vi "KH_DAQ_TURCK_ScaleAI.vi"(8 "Messwert Turck":i16[](array[numeric]), 10 "EIP_AI":T1 {"Offset" format="%.4f"; "Phys Max" format="%.4f"; "Phys Min" format="%.4f"}, 11 "Nr.":i32) -> (3 "Messwert skaliert":sgl[](array[numeric]))   [LabVIEW 2021]
uses:
  KH_DAQ_TypeDefs_Cluster AI.ctl
  KH_DAQ_TypeDefs_Messbereich.ctl
  KH EthernetIPConfig 17.14/KH EthernetIPConfig TypeDefs ModuleTyp.ctl
  KH_DAQ_TypeDefs_Bereich.ctl
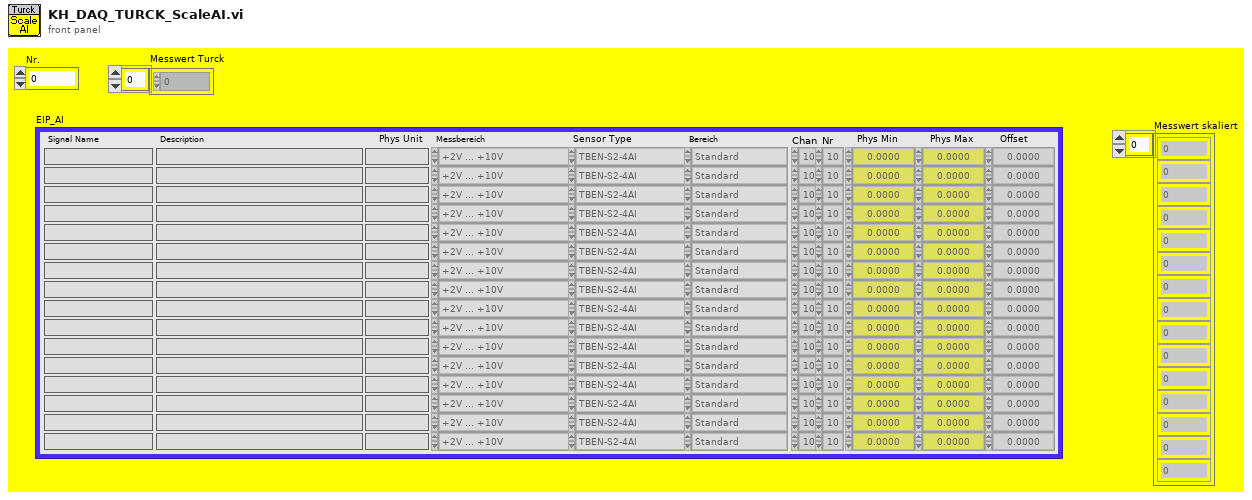
[diagram p1: front panel]
types:
  T1 = typedef "KH_DAQ_TypeDefs_Cluster AI.ctl" = cluster{"Signal Name":string[], "Description":string[], "Phys Unit":string[], "Messbereich":T2[], "Chan":u16[], "Phys Min":sgl[], "Phys Max":sgl[], "Offset":sgl[], "Nr":u16[], "SensorType 2":T3[], "Bereich":T4[]}
  T2 = typedef "KH_DAQ_TypeDefs_Messbereich.ctl" = enum16{"-10V ... +10V", "0V ... +10V", "+2V ... +10V", "0V ... +5V", "+1V ... +5V", "-1V ... +1V", "-500mV ... +500mV", "-100mV ... +100mV", "-50mV ... +50mV", "0mA ... +20mA", "+4mA ... +20mA", "-20mA ... +20mA", "0 Ohm ... 100 Ohm", "0 Ohm ... 400 Ohm", "0 Ohm ... 2000 Ohm", "0 Ohm ... 4000 Ohm", "-200°C ... 150°C PT100", "-200°C ... 150°C PT200", "-200°C ... 150°C PT500", "-200°C ... 150°C PT1000", "-60°C ... 150°C Ni100", "-60°C ... 150°C Ni1000", "-200°C ... 850°C PT100", "-200°C ... 850°C PT200", "-200°C ... 850°C PT500", "-200°C ... 850°C PT1000", "-50°C ... 250°C Ni100", "-50°C ... 250° Ni 1000"}
  T3 = typedef "KH EthernetIPConfig TypeDefs ModuleTyp.ctl" = enum16{"TBEN-S2-4AI", "TBEN-S1-8DXP", "TBEN-S2-2RFID-4DXP", "TBEN-S2-4AO", "TBEN-S2-4IOL"}
  T4 = typedef "KH_DAQ_TypeDefs_Bereich.ctl" = enum16{"Standard", "extended Range", "NE43", ""}
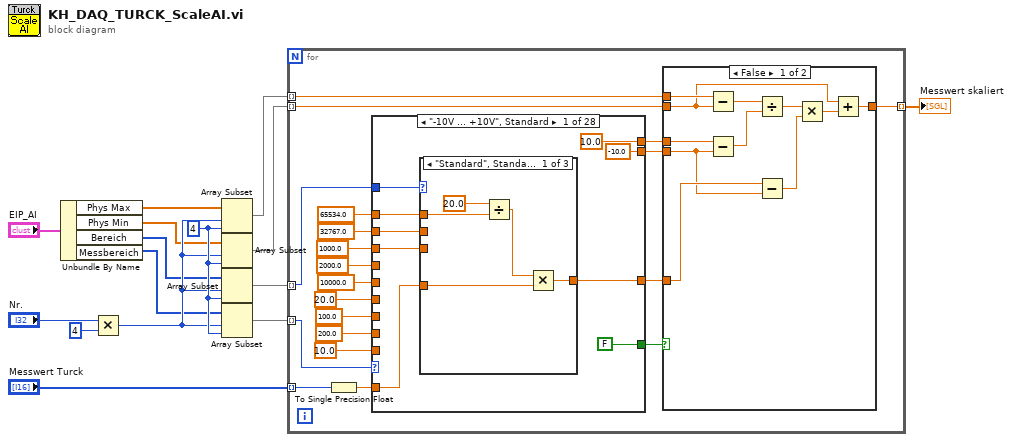
[diagram p0: block diagram]
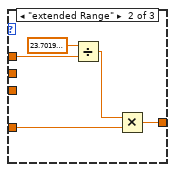
[diagram p3: hidden frame]
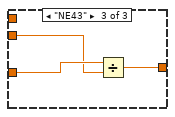
[diagram p4: hidden frame]
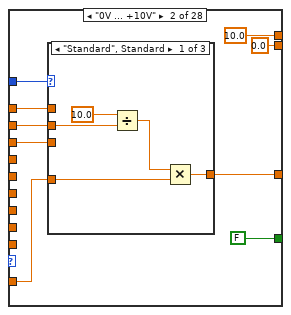
[diagram p5: hidden frame]
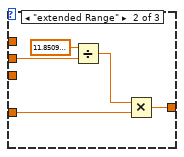
[diagram p6: hidden frame]
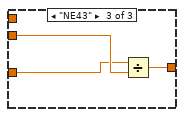
[diagram p7: hidden frame]
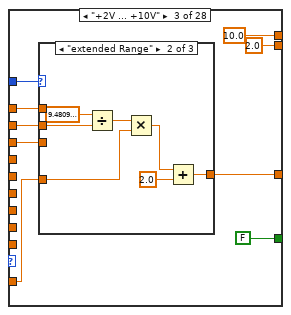
[diagram p8: hidden frame]
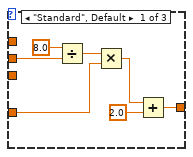
[diagram p9: hidden frame]
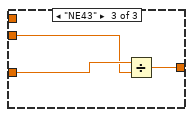
[diagram p10: hidden frame]
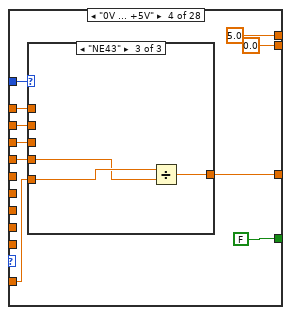
[diagram p11: hidden frame]
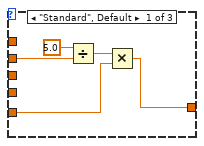
[diagram p12: hidden frame]
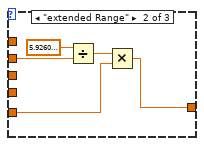
[diagram p13: hidden frame]
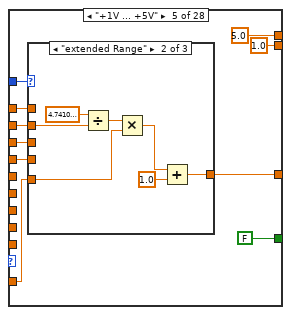
[diagram p14: hidden frame]
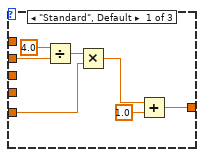
[diagram p15: hidden frame]
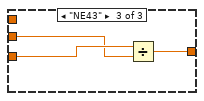
[diagram p16: hidden frame]
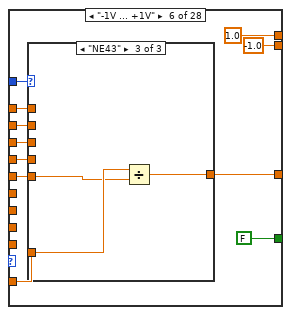
[diagram p17: hidden frame]
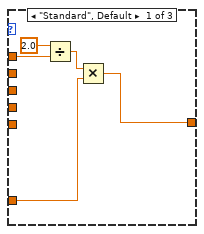
[diagram p18: hidden frame]
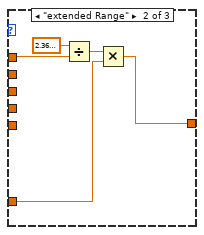
[diagram p19: hidden frame]
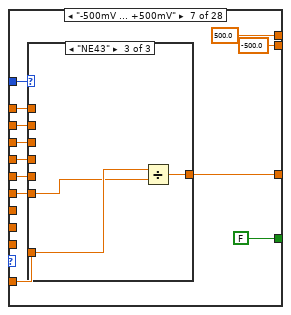
[diagram p20: hidden frame]
diagram:
  w15 = 4 ("length")
  n1 = Unbundle By Name("EIP_AI") -> ("Phys Max"=w8:sgl[], "Phys Min"=w9:sgl[], "Bereich"=w10:T4[], "Messbereich"=w11:T2[])
  n2 = Multiply(x="Nr.", y=4) -> (x*y=w14:i32)
  n3 = Array Subset(array=w8, index=w14, length=w15) -> (w7:sgl[])
  n4 = Array Subset(array=w9, index=w14, length=w15) -> (w6:sgl[])
  n5 = Array Subset(array=w10, index=w14, length=w15) -> (w5:T4[])
  n6 = Array Subset(array=w11, index=w14, length=w15) -> (w4:T2[])
  n7 = for {
    tunnel: [w22] -> w1 mode=indexing
    tunnel: w7 -> [w20] mode=indexing
    tunnel: w6 -> [w19] mode=indexing
    tunnel: w5 -> [w18] mode=indexing
    tunnel: w4 -> [w17] mode=indexing
    tunnel: "Messwert Turck" -> [w16] mode=indexing
    n8 = To Single Precision Float(number=w16) -> (single precision float=w32:sgl)
    n9 = case shown="\"-10V ... +10V\", Standard" w17 {
      tunnel: w18 -> [w56 w78 w100 w127 w150 w178 w203 w229 w256 w283 w310 w341 _ _ _ _ _ _ _ _ _ _ _ _ _ _ _ _]
      tunnel: sgl 65534.0 ("Sollwert 2") -> [w55 w77 w99 w126 w149 w177 w202 w228 w255 w282 w309 w340 _ _ _ _ _ _ _ _ _ _ _ _ _ _ _ _]
      tunnel: sgl 32767.0 ("Sollwert 2") -> [w54 w76 w98 w125 w148 w176 w201 w227 w254 w281 w308 w339 w362 w370 w378 w386 _ _ _ _ _ _ _ _ _ _ _ _]
      tunnel: sgl 1000.0 ("Sollwert 2") -> [w53 w75 w97 w124 w147 w175 w200 w226 w253 w280 w307 w338 _ _ _ _ _ _ _ _ _ _ _ _ _ _ _ _]
      tunnel: w32 -> [w52 w74 w96 w123 w146 w174 w199 w225 w252 w279 w306 w337 w361 w369 w377 w385 w390 w394 w398 w402 w406 w410 w414 w418 w422 w426 w430 w434]
      tunnel: [w51 w73 w95 w122 w145 w173 w198 w224 w251 w278 w305 w336 w360 w368 w376 w384 w389 w393 w397 w401 w405 w409 w412 w417 w421 w425 w429 w433] -> w23
      tunnel: sgl 2000.0 ("Sollwert 2") -> [_ _ _ w121 w144 w172 w197 w223 w250 w277 w304 w335 _ _ _ _ _ _ _ _ _ _ _ _ _ _ _ _]
      tunnel: sgl 10000.0 ("Sollwert 2") -> [_ _ _ _ _ w171 w196 w222 w249 w276 w303 w334 _ _ _ _ _ _ _ _ _ _ _ _ _ _ _ _]
      tunnel: sgl 20.0 ("Sollwert 2") -> [_ _ _ _ _ _ w195 w221 w248 w275 w302 w333 _ _ _ _ _ _ _ _ _ _ _ _ _ _ _ _]
      tunnel: sgl 100.0 ("Sollwert 2") -> [_ _ _ _ _ _ _ w220 w247 w274 w301 w332 _ _ _ _ w388 w392 w396 w400 w404 w408 _ _ _ _ _ _]
      tunnel: sgl 200.0 ("Sollwert 2") -> [_ _ _ _ _ _ _ _ w246 w273 w300 w331 _ _ _ _ _ _ _ _ _ _ _ _ _ _ _ _]
      tunnel: sgl 10.0 ("Sollwert 2") -> [_ _ _ _ _ _ _ _ _ _ _ _ _ _ _ _ _ _ _ _ _ _ w413 w416 w420 w424 w428 w432]
      tunnel: [sgl -10.0 ("Messwert 2") sgl 0.0 ("Messwert 2") sgl 2.0 ("Messwert 2") sgl 0.0 ("Messwert 2") sgl 1.0 ("Messwert 2") sgl -1.0 ("Messwert 2") sgl -500.0 ("Messwert 2") sgl -100.0 ("Messwert 2") sgl -50.0 ("Messwert 2") sgl 0.0 ("Messwert 2") sgl 4.0 ("Messwert 2") sgl -20.0 ("Messwert 2") sgl 0.0 ("Messwert 2") sgl 0.0 ("Messwert 2") sgl 0.0 ("Messwert 2") sgl 0.0 ("Messwert 2") _ _ _ _ _ _ _ _ _ _ _ _] -> w25
      tunnel: [sgl 10.0 ("Messwert 2") sgl 10.0 ("Messwert 2") sgl 10.0 ("Messwert 2") sgl 5.0 ("Messwert 2") sgl 5.0 ("Messwert 2") sgl 1.0 ("Messwert 2") sgl 500.0 ("Messwert 2") sgl 100.0 ("Messwert 2") sgl 50.0 ("Messwert 2") sgl 20.0 ("Messwert 2") sgl 20.0 ("Messwert 2") sgl 20.0 ("Messwert 2") sgl 100.0 ("Messwert 2") sgl 400.0 ("Messwert 2") sgl 2000.0 ("Messwert 2") sgl 4000.0 ("Messwert 2") _ _ _ _ _ _ _ _ _ _ _ _] -> w24
      tunnel: [FALSE FALSE FALSE FALSE FALSE FALSE FALSE FALSE FALSE FALSE FALSE FALSE FALSE FALSE FALSE FALSE TRUE TRUE TRUE TRUE TRUE TRUE TRUE TRUE TRUE TRUE TRUE TRUE] -> w21
      frame "-10V ... +10V", Default {
        n10 = case shown="\"Standard\", Standard" w56 {
          tunnel: w55 -> [w60 w65 _]
          tunnel: w54 -> [_ _ _]
          tunnel: w53 -> [_ _ w68]
          tunnel: w52 -> [w59 w64 w69]
          tunnel: [w57 w62 w67] -> w51
          frame "Standard", Default {
            n11 = Divide(x=sgl 20.0 ("Messwert 2"), y=w60) -> (x/y=w58:sgl)
            n12 = Multiply(x=w58, y=w59) -> (x*y=w57:sgl)
          }
          frame "extended Range" {
            n13 = Divide(x=sgl 23.702 ("Messwert 2"), y=w65) -> (x/y=w63:sgl)
            n14 = Multiply(x=w63, y=w64) -> (x*y=w62:sgl)
          }
          frame "NE43" {
            n15 = Divide(x=w69, y=w68) -> (x/y=w67:sgl)
          }
        }
      }
      frame "0V ... +10V" {
        n16 = case shown="\"Standard\", Standard" w78 {
          tunnel: w77 -> [_ _ _]
          tunnel: w76 -> [w79 w84 _]
          tunnel: w75 -> [_ _ w91]
          tunnel: w74 -> [w82 w87 w90]
          tunnel: [w80 w85 w89] -> w73
          frame "Standard", Default {
            n17 = Divide(x=sgl 10.0 ("Messwert 2"), y=w79) -> (x/y=w81:sgl)
            n18 = Multiply(x=w81, y=w82) -> (x*y=w80:sgl)
          }
          frame "extended Range" {
            n19 = Divide(x=sgl 11.851 ("Messwert 2"), y=w84) -> (x/y=w86:sgl)
            n20 = Multiply(x=w86, y=w87) -> (x*y=w85:sgl)
          }
          frame "NE43" {
            n21 = Divide(x=w90, y=w91) -> (x/y=w89:sgl)
          }
        }
      }
      frame "+2V ... +10V" {
        n22 = case shown="\"extended Range\"" w100 {
          tunnel: w99 -> [_ _ _]
          tunnel: w98 -> [w104 w111 _]
          tunnel: w97 -> [_ _ w116]
          tunnel: w96 -> [w106 w113 w117]
          tunnel: [w103 w110 w115] -> w95
          frame "Standard", Default {
            n23 = Divide(x=sgl 8.0 ("Messwert 2"), y=w104) -> (x/y=w105:sgl)
            n24 = Multiply(x=w105, y=w106) -> (x*y=w102:sgl)
            n25 = Add(x=w102, y=sgl 2.0) -> (x+y=w103:sgl)
          }
          frame "extended Range" {
            n26 = Divide(x=sgl 9.481 ("Messwert 2"), y=w111) -> (x/y=w112:sgl)
            n27 = Multiply(x=w112, y=w113) -> (x*y=w109:sgl)
            n28 = Add(x=w109, y=sgl 2.0) -> (x+y=w110:sgl)
          }
          frame "NE43" {
            n29 = Divide(x=w117, y=w116) -> (x/y=w115:sgl)
          }
        }
      }
      frame "0V ... +5V" {
        n30 = case shown="\"NE43\"" w127 {
          tunnel: w126 -> [_ _ _]
          tunnel: w125 -> [w129 w134 _]
          tunnel: w124 -> [_ _ _]
          tunnel: w123 -> [w131 w136 w140]
          tunnel: [w128 w133 w138] -> w122
          tunnel: w121 -> [_ _ w139]
          frame "Standard", Default {
            n31 = Divide(x=sgl 5.0 ("Messwert 2"), y=w129) -> (x/y=w130:sgl)
            n32 = Multiply(x=w130, y=w131) -> (x*y=w128:sgl)
          }
          frame "extended Range" {
            n33 = Divide(x=sgl 5.926 ("Messwert 2"), y=w134) -> (x/y=w135:sgl)
            n34 = Multiply(x=w135, y=w136) -> (x*y=w133:sgl)
          }
          frame "NE43" {
            n35 = Divide(x=w140, y=w139) -> (x/y=w138:sgl)
          }
        }
      }
      frame "+1V ... +5V" {
        n36 = case shown="\"extended Range\"" w150 {
          tunnel: w149 -> [_ _ _]
          tunnel: w148 -> [w154 w161 _]
          tunnel: w147 -> [_ _ _]
          tunnel: w146 -> [w156 w163 w166]
          tunnel: [w152 w159 w167] -> w145
          tunnel: w144 -> [_ _ w165]
          frame "Standard", Default {
            n37 = Divide(x=sgl 4.0 ("Messwert 2"), y=w154) -> (x/y=w155:sgl)
            n38 = Multiply(x=w155, y=w156) -> (x*y=w153:sgl)
            n39 = Add(x=w153, y=sgl 1.0) -> (x+y=w152:sgl)
          }
          frame "extended Range" {
            n40 = Divide(x=sgl 4.741 ("Messwert 2"), y=w161) -> (x/y=w162:sgl)
            n41 = Multiply(x=w162, y=w163) -> (x*y=w158:sgl)
            n42 = Add(x=w158, y=sgl 1.0) -> (x+y=w159:sgl)
          }
          frame "NE43" {
            n43 = Divide(x=w166, y=w165) -> (x/y=w167:sgl)
          }
        }
      }
      frame "-1V ... +1V" {
        n44 = case shown="\"NE43\"" w178 {
          tunnel: w177 -> [w180 w185 _]
          tunnel: w176 -> [_ _ _]
          tunnel: w175 -> [_ _ _]
          tunnel: w174 -> [w182 w187 w191]
          tunnel: [w179 w184 w189] -> w173
          tunnel: w172 -> [_ _ _]
          tunnel: w171 -> [_ _ w190]
          frame "Standard", Default {
            n45 = Divide(x=sgl 2.0 ("Messwert 2"), y=w180) -> (x/y=w181:sgl)
            n46 = Multiply(x=w181, y=w182) -> (x*y=w179:sgl)
          }
          frame "extended Range" {
            n47 = Divide(x=sgl 2.37 ("Messwert 2"), y=w185) -> (x/y=w186:sgl)
            n48 = Multiply(x=w186, y=w187) -> (x*y=w184:sgl)
          }
          frame "NE43" {
            n49 = Divide(x=w191, y=w190) -> (x/y=w189:sgl)
          }
        }
      }
      frame "-500mV ... +500mV" {
        n50 = case shown="\"NE43\"" w203 {
          tunnel: w202 -> [w205 w210 _]
          tunnel: w201 -> [_ _ _]
          tunnel: w200 -> [_ _ _]
          tunnel: w199 -> [w207 w212 w215]
          tunnel: [w204 w209 w216] -> w198
          tunnel: w197 -> [_ _ _]
          tunnel: w196 -> [_ _ _]
          tunnel: w195 -> [_ _ w214]
          frame "Standard", Default {
            n51 = Divide(x=sgl 1000.0 ("Messwert 2"), y=w205) -> (x/y=w206:sgl)
            n52 = Multiply(x=w206, y=w207) -> (x*y=w204:sgl)
          }
          frame "extended Range" {
            n53 = Divide(x=sgl 1185.2 ("Messwert 2"), y=w210) -> (x/y=w211:sgl)
            n54 = Multiply(x=w211, y=w212) -> (x*y=w209:sgl)
          }
          frame "NE43" {
            n55 = Divide(x=w215, y=w214) -> (x/y=w216:sgl)
          }
        }
      }
      frame "-100mV ... +100mV" {
        n56 = case shown="\"NE43\"" w229 {
          tunnel: w228 -> [w231 w236 _]
          tunnel: w227 -> [_ _ _]
          tunnel: w226 -> [_ _ _]
          tunnel: w225 -> [w233 w238 w241]
          tunnel: [w230 w235 w242] -> w224
          tunnel: w223 -> [_ _ _]
          tunnel: w222 -> [_ _ _]
          tunnel: w221 -> [_ _ _]
          tunnel: w220 -> [_ _ w240]
          frame "Standard", Default {
            n57 = Divide(x=sgl 200.0 ("Messwert 2"), y=w231) -> (x/y=w232:sgl)
            n58 = Multiply(x=w232, y=w233) -> (x*y=w230:sgl)
          }
          frame "extended Range" {
            n59 = Divide(x=sgl 237.0 ("Messwert 2"), y=w236) -> (x/y=w237:sgl)
            n60 = Multiply(x=w237, y=w238) -> (x*y=w235:sgl)
          }
          frame "NE43" {
            n61 = Divide(x=w241, y=w240) -> (x/y=w242:sgl)
          }
        }
      }
      frame "-50mV ... +50mV" {
        n62 = case shown="\"NE43\"" w256 {
          tunnel: w255 -> [w258 w263 _]
          tunnel: w254 -> [_ _ _]
          tunnel: w253 -> [_ _ _]
          tunnel: w252 -> [w260 w265 w268]
          tunnel: [w257 w262 w269] -> w251
          tunnel: w250 -> [_ _ _]
          tunnel: w249 -> [_ _ _]
          tunnel: w248 -> [_ _ _]
          tunnel: w247 -> [_ _ _]
          tunnel: w246 -> [_ _ w267]
          frame "Standard", Default {
            n63 = Divide(x=sgl 100.0 ("Messwert 2"), y=w258) -> (x/y=w259:sgl)
            n64 = Multiply(x=w259, y=w260) -> (x*y=w257:sgl)
          }
          frame "extended Range" {
            n65 = Divide(x=sgl 118.6 ("Messwert 2"), y=w263) -> (x/y=w264:sgl)
            n66 = Multiply(x=w264, y=w265) -> (x*y=w262:sgl)
          }
          frame "NE43" {
            n67 = Divide(x=w268, y=w267) -> (x/y=w269:sgl)
          }
        }
      }
      frame "0mA ... +20mA" {
        n68 = case shown="\"Standard\", Standard" w283 {
          tunnel: w282 -> [_ _ _]
          tunnel: w281 -> [w284 w289 _]
          tunnel: w280 -> [_ _ w294]
          tunnel: w279 -> [w287 w292 w295]
          tunnel: [w285 w290 w296] -> w278
          tunnel: w277 -> [_ _ _]
          tunnel: w276 -> [_ _ _]
          tunnel: w275 -> [_ _ _]
          tunnel: w274 -> [_ _ _]
          tunnel: w273 -> [_ _ _]
          frame "Standard", Default {
            n69 = Divide(x=sgl 20.0 ("Messwert 2"), y=w284) -> (x/y=w286:sgl)
            n70 = Multiply(x=w286, y=w287) -> (x*y=w285:sgl)
          }
          frame "extended Range" {
            n71 = Divide(x=sgl 23.703 ("Messwert 2"), y=w289) -> (x/y=w291:sgl)
            n72 = Multiply(x=w291, y=w292) -> (x*y=w290:sgl)
          }
          frame "NE43" {
            n73 = Divide(x=w295, y=w294) -> (x/y=w296:sgl)
          }
        }
      }
      frame "+4mA ... +20mA" {
        n74 = case shown="\"extended Range\"" w310 {
          tunnel: w309 -> [_ _ _]
          tunnel: w308 -> [w314 w321 _]
          tunnel: w307 -> [_ _ w325]
          tunnel: w306 -> [w316 w323 w326]
          tunnel: [w313 w320 w327] -> w305
          tunnel: w304 -> [_ _ _]
          tunnel: w303 -> [_ _ _]
          tunnel: w302 -> [_ _ _]
          tunnel: w301 -> [_ _ _]
          tunnel: w300 -> [_ _ _]
          frame "Standard", Default {
            n75 = Divide(x=sgl 16.0 ("Messwert 2"), y=w314) -> (x/y=w315:sgl)
            n76 = Multiply(x=w315, y=w316) -> (x*y=w312:sgl)
            n77 = Add(x=w312, y=sgl 4.0) -> (x+y=w313:sgl)
          }
          frame "extended Range" {
            n78 = Divide(x=sgl 18.962 ("Messwert 2"), y=w321) -> (x/y=w322:sgl)
            n79 = Multiply(x=w322, y=w323) -> (x*y=w319:sgl)
            n80 = Add(x=w319, y=sgl 4.0) -> (x+y=w320:sgl)
          }
          frame "NE43" {
            n81 = Divide(x=w326, y=w325) -> (x/y=w327:sgl)
          }
        }
      }
      frame "-20mA ... +20mA" {
        n82 = case shown="\"NE43\"" w341 {
          tunnel: w340 -> [_ _ _]
          tunnel: w339 -> [w343 w348 _]
          tunnel: w338 -> [_ _ w352]
          tunnel: w337 -> [w345 w350 w353]
          tunnel: [w342 w347 w354] -> w336
          tunnel: w335 -> [_ _ _]
          tunnel: w334 -> [_ _ _]
          tunnel: w333 -> [_ _ _]
          tunnel: w332 -> [_ _ _]
          tunnel: w331 -> [_ _ _]
          frame "Standard", Default {
            n83 = Divide(x=sgl 40.0 ("Messwert 2"), y=w343) -> (x/y=w344:sgl)
            n84 = Multiply(x=w344, y=w345) -> (x*y=w342:sgl)
          }
          frame "extended Range" {
            n85 = Divide(x=sgl 47.406 ("Messwert 2"), y=w348) -> (x/y=w349:sgl)
            n86 = Multiply(x=w349, y=w350) -> (x*y=w347:sgl)
          }
          frame "NE43" {
            n87 = Divide(x=w353, y=w352) -> (x/y=w354:sgl)
          }
        }
      }
      frame "0 Ohm ... 100 Ohm" {
        n88 = Divide(x=sgl 100.0 ("Messwert 2"), y=w362) -> (x/y=w358:sgl)
        n89 = Multiply(x=w358, y=w361) -> (x*y=w360:sgl)
      }
      frame "0 Ohm ... 400 Ohm" {
        n90 = Divide(x=sgl 400.0 ("Messwert 2"), y=w370) -> (x/y=w366:sgl)
        n91 = Multiply(x=w366, y=w369) -> (x*y=w368:sgl)
      }
      frame "0 Ohm ... 2000 Ohm" {
        n92 = Divide(x=sgl 2000.0 ("Messwert 2"), y=w378) -> (x/y=w374:sgl)
        n93 = Multiply(x=w374, y=w377) -> (x*y=w376:sgl)
      }
      frame "0 Ohm ... 4000 Ohm" {
        n94 = Divide(x=sgl 4000.0 ("Messwert 2"), y=w386) -> (x/y=w382:sgl)
        n95 = Multiply(x=w382, y=w385) -> (x*y=w384:sgl)
      }
      frame "-200°C ... 150°C PT100" {
        n96 = Divide(x=w390, y=w388) -> (x/y=w389:sgl)
      }
      frame "-200°C ... 150°C PT200" {
        n97 = Divide(x=w394, y=w392) -> (x/y=w393:sgl)
      }
      frame "-200°C ... 150°C PT500" {
        n98 = Divide(x=w398, y=w396) -> (x/y=w397:sgl)
      }
      frame "-200°C ... 150°C PT1000" {
        n99 = Divide(x=w402, y=w400) -> (x/y=w401:sgl)
      }
      frame "-60°C ... 150°C Ni100" {
        n100 = Divide(x=w406, y=w404) -> (x/y=w405:sgl)
      }
      frame "-60°C ... 150°C Ni1000" {
        n101 = Divide(x=w410, y=w408) -> (x/y=w409:sgl)
      }
      frame "-200°C ... 850°C PT100" {
        n102 = Divide(x=w414, y=w413) -> (x/y=w412:sgl)
      }
      frame "-200°C ... 850°C PT200" {
        n103 = Divide(x=w418, y=w416) -> (x/y=w417:sgl)
      }
      frame "-200°C ... 850°C PT500" {
        n104 = Divide(x=w422, y=w420) -> (x/y=w421:sgl)
      }
      frame "-200°C ... 850°C PT1000" {
        n105 = Divide(x=w426, y=w424) -> (x/y=w425:sgl)
      }
      frame "-50°C ... 250°C Ni100" {
        n106 = Divide(x=w430, y=w428) -> (x/y=w429:sgl)
      }
      frame "-50°C ... 250° Ni 1000" {
        n107 = Divide(x=w434, y=w432) -> (x/y=w433:sgl)
      }
    }
    n108 = case shown="False" w21 {
      tunnel: [w41 w47] -> w22
      tunnel: w23 -> [w40 w47]
      tunnel: w20 -> [w39 _]
      tunnel: w19 -> [w38 _]
      tunnel: w25 -> [w37 _]
      tunnel: w24 -> [w36 _]
      frame False {
        n109 = Subtract(x=w39, y=w38) -> (x-y=w46:sgl)
        n110 = Subtract(x=w36, y=w37) -> (x-y=w45:sgl)
        n111 = Divide(x=w46, y=w45) -> (x/y=w44:sgl)
        n112 = Subtract(x=w40, y=w37) -> (x-y=w43:sgl)
        n113 = Multiply(x=w44, y=w43) -> (x*y=w42:sgl)
        n114 = Add(x=w38, y=w42) -> (x+y=w41:sgl)
      }
      frame True {
      }
    }
  }
  "Messwert skaliert" <- w1
